vi "BasisFunctions.vi"(6 "Basis Set":u16(ring)=1 items=["Fourier", "Tents", "Blocks"], 9 "Window Length (s)":dbl=12.0, 10 "Number of Basis Functions":i32=8, 11 "dt":dbl) -> (3 "Array of Basis Functions":dbl[][](array[numeric]))   [LabVIEW 2013]
uses:
  <vilib>/Analysis/1siggen.llb/General Aperiodic Triangle.vi
  <vilib>/Analysis/NI_AALBase.lvlib
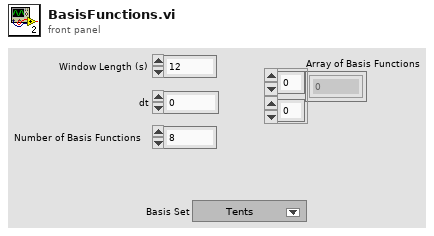
[diagram p1: front panel]
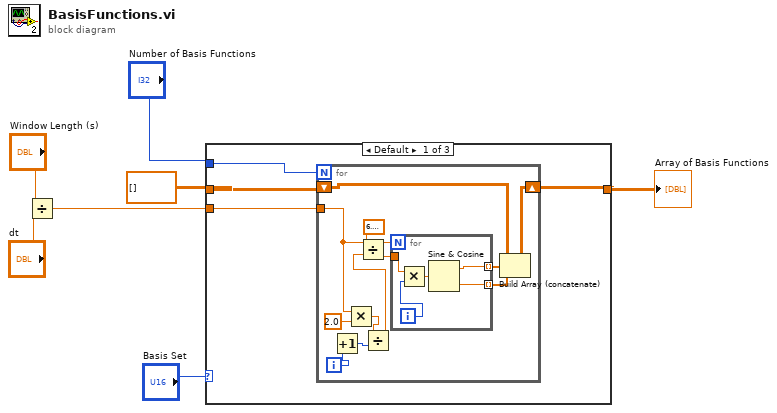
[diagram p0: block diagram]
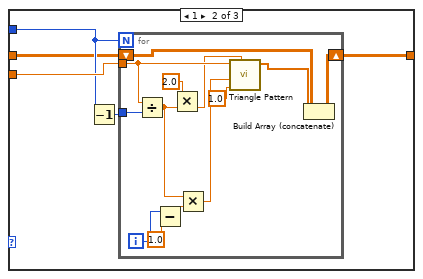
[diagram p2: hidden frame]
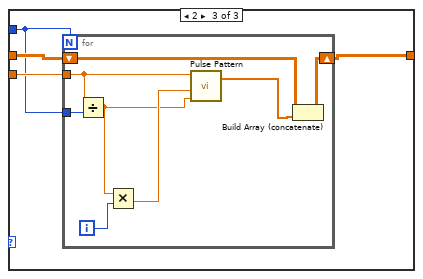
[diagram p3: hidden frame]
diagram:
  n1 = Divide(x="Window Length (s)", y="dt") -> (x/y=w3:dbl)
  n2 = case shown="Default" "Basis Set" {
    tunnel: w3 -> [w11 w33 w50]
    tunnel: "Number of Basis Functions" -> [w8 w30 w47]
    tunnel: [w10 w32 w49] -> w7
    tunnel: dbl[][] [] -> [w9 w29 w48]
    frame Default {
      n3 = for {
        N: w8 -> [_]
        tunnel: w11 -> [w19]
        shift-right: [w14] -> w10
        shift-left: w9 -> [w13]
        i -> [w12]
        n4 = Increment(x=w12) -> (x+1=w15:i32)
        n5 = Multiply(x=w19, y=2.0) -> (x*y=w17:dbl)
        n6 = Divide(x=w17, y=w15) -> (x/y=w16:dbl)
        n7 = Divide(x=6.283185307179586, y=w16) -> (x/y=w22:dbl)
        n8 = for {
          N: w19 -> [_]
          tunnel: [w28] -> w21 mode=indexing
          tunnel: [w27] -> w20 mode=indexing
          tunnel: w22 -> [w24]
          i -> [w25]
          n9 = Multiply(x=w24, y=w25) -> (x*y=w26:dbl)
          n10 = Sine & Cosine(0:w26) -> (1:w28:dbl, 2:w27:dbl)
        }
        n11 = Build Array (concatenate)(w13, w21, w20) -> (w14:dbl[][])
      }
    }
    frame 1 {
      n12 = Decrement(x=w30) -> (x-1=w31:i32)
      n13 = for {
        N: w30 -> [_]
        tunnel: w31 -> [w46]
        tunnel: w33 -> [w45]
        shift-right: [w36] -> w32
        shift-left: w29 -> [w37]
        i -> [w35]
        n14 = Divide(x=w45, y=w46) -> (x/y=w38:dbl)
        n15 = Subtract(x=w35, y=1.0) -> (x-y=w41:dbl)
        n16 = Multiply(x=2.0, y=w38) -> (x*y=w39:dbl)
        n17 = Multiply(x=w38, y=w41) -> (x*y=w42:dbl)
        n18 = call <vilib>:"Triangle Pattern.vi"("width (s)"=w39, "delta t (s)"=1.0, "delay (s)"=w42, "samples"=w45) -> ("Triangle Pattern"=w34:dbl[])  [unwired: 6 in, 1 out]
        n19 = Build Array (concatenate)(w37, w34) -> (w36:dbl[][])
      }
    }
    frame 2 {
      n20 = for {
        N: w47 -> [_]
        tunnel: w47 -> [w58]
        tunnel: w50 -> [w52]
        shift-right: [w56] -> w49
        shift-left: w48 -> [w55]
        i -> [w57]
        n21 = Divide(x=w52, y=w58) -> (x/y=w53:dbl)
        n22 = Multiply(x=w53, y=w57) -> (x*y=w54:dbl)
        n23 = call <vilib>:"Pulse Pattern.vi"("width"=w53, "delay"=w54, "samples"=w52) -> ("Pulse Pattern"=w51:dbl[])  [unwired: 1 in, 1 out]
        n24 = Build Array (concatenate)(w55, w51) -> (w56:dbl[][])
      }
    }
  }
  "Array of Basis Functions" <- w7
